vi "Dialog_parameters (SubVI).vi"() -> (3 "Cancelled?":bool)   [LabVIEW 2017]
doc: "Use this template to create a dialog box with event handling."
uses:
  Global_SNK3_HF.vi
  E:/_git/LV_Unicorn/LV_Unicorn.lvlib
panel:
  in  "TimerSyncInt":i32=10000 caption="Частота следования тактов, Гц" min=1000 max=100000
  in  "Meas":bool=TRUE
  in  "Tab2":T1(tab)
  in  "EncoderSync":i64=1 caption="Величина \"К\""
  out "NumOfRuns":i32=994875 caption="Счетчик количества запусков цикла"
  in  "DataEncodersParam2":enum16{"Encoder1CurrData", "PulseCurrData"}(ring) caption="Параметры поля \"Encoders Param 2\""
  in  "EncoderNum":u16(ring)=1 caption="Номер энкодера для режима \"Энкодер\"" items=["1"=1, "2"=2]
  in  "SyncMode":u16(ring)=1 caption="Источник синхронизации" items=["Внутренний таймер"=1, "Энкодер"=2, "Внешний импульс"=3]
  in  "DataEncodersParam1":enum16{"Encoder1CurrData", "PulseCurrData"}(ring) caption="Параметры поля \"Encoders Param 1\""
  in  "Encoder2CurrData":i64 caption="Текущее значение счетчика энкодера 2"
  in  "Encoder2ScalingFactor":i32=100 caption="Масштабный коэффициент, нм/имп"
  in  "Encoder2AInv":bool
  in  "Encoder2BInv":bool
  in  "Encoder2ZInv":bool
  in  "Encoder2ZEn":bool
  in  "Encoder2En":bool
  in  "Encoder1CurrData":i64 caption="Текущее значение счетчика энкодера 1"
  in  "Encoder1ScalingFactor":i32=100 caption="Масштабный коэффициент, нм/имп"
  in  "Encoder1AInv":bool
  in  "Encoder1BInv":bool
  in  "Encoder1ZInv":bool
  in  "Encoder1ZEn":bool
  in  "Encoder1En":bool
  in  "PulseCurrData":i64 caption="Текущее значение счетчика импульсов"
  in  "PulseSensitivity":u16(ring)=1 caption="Тип запуска для режима" items=["Фронт"=1, "Срез"=2, "Оба"=3]
  in  "PulseScalingFactor":i32=100 caption="Масштабный коэффициент, нм/имп" min=0
  in  "PulseInput":T2(ring) caption="Вход импульса запуска"
  in  "PulseCounterEn":bool
  in  "FPGA1ExtRAMBuffEn":bool=TRUE
  in  "FPGA0ExtRAMBuffEn":bool=TRUE
  in  "IPEn50Om":bool caption="Демпфирование ПЭП(50 Ом)"
  in  "ReceiverStaticGainParam":T3(ring) caption="Коэфф усиления приемников"
  in  "SaveParam":bool
  out "IPAddressCur":string caption="Текущий IP адрес ЭБ"
  in  "IPDefaultNetMask":string caption="Маска подсети"
  in  "IPDefaultGW":string caption="Основной шлюз"
  in  "IPDefaultAddress":string caption="IP адрес электронного блока по умолчанию"
  in  "IPAddressUDP":string caption="IP адрес для передачи UPD пакетов"
  in  "Port1UDP":u16 caption="Порт для передачи UPD пакетов с разъемов X1...X8"
  in  "Port2UDP":u16 caption="Порт для передачи UPD пакетов с разъемов X9...X16"
  in  "Cancel":bool
  in  "OK":bool
  # "Энкодер 1"
  # "Энкодер 2"
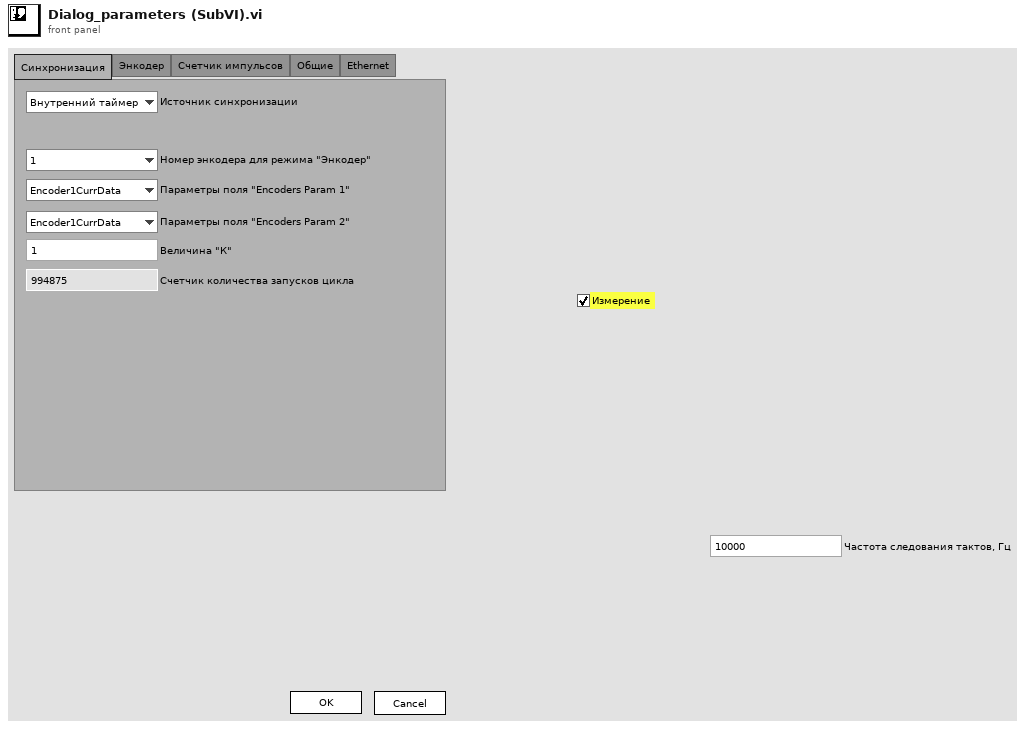
[diagram p1: front panel]
types:
  T1 = enum32{"Синхронизация", "Энкодер", "Счетчик импульсов", "Общие", "Ethernet"}
  T2 = enum16{"X17 вход 1", "X17 вход 2", "X17 вход 3", "X18 вход 1", "X18 вход 2", "X18 вход 3"}
  T3 = enum16{"Коэф. усил., дБ", "Вых. ЦАП (10 бит)", "Вых. ЦАП "}
  T4 = typedef "LV_Unicorn.lvlib/unicorn_Param.ctl" = cluster{"conParam":T5, "Param":T6}
  T5 = typedef "LV_Unicorn.lvlib/unicorn_conn.ctl" = cluster{"ReadIntParam":bool, "ReadDescrParam":bool, "ReadFloatParam":bool, "debug":bool, "ReadJSON":bool, "IP_address":string, "N_attempts":i32, "type_con":enum16{"Serial", "TCP"}, "MB_address":i32, "VISA":refnum<visa-resource-name>, "connection ID":refnum<k5>, "nameDevices":string, "timeout":i32, "port":u16, "type_version":string, "baud_rate":u32, "VersionControl":bool, "TCP_conn":bool, "WindowSize":i32}
  T6 = typedef "LV_Unicorn.lvlib/unicorn_JSON.ctl" = cluster{"NumParam":cluster{"NTelem":i32, "NInt":i32, "NFloat":i32, "NTable":i32}, "ParamInt":T7, "Telemetry":T8, "Table":T9, "ParamFloat":T10}
  T7 = typedef "LV_Unicorn.lvlib/unicorn_ParamInt.ctl" = cluster{"ID":string, "Num":i32, "Name":string, "Type":string, "Enum":string, "Desc":string, "Unit":string, "Access":string, "FormatStr":string, "Min":i32, "Max":i32}[]
  T8 = typedef "LV_Unicorn.lvlib/unicorn_Telemetry.ctl" = cluster{"ID":string, "Num":i32, "Name":string, "Desc":string, "Unit":string, "FormatStr":string, "Min":i32, "Max":i32}[]
  T9 = typedef "LV_Unicorn.lvlib/unicorn_Table.ctl" = cluster{"Num":i32, "Access":string, "ColumnCount":i32, "NeedParamPrepare":bool, "Columns":cluster{"Column":i32, "Desc":string, "Name":string}[], "DataType":string, "FormatStr":string, "ID":string, "Name":string, "RowCount":i32, "Rows":cluster{"Desc":string, "ID":string, "Max":i32, "Min":i32, "Name":string, "Row":i32, "Unit":string}[], "Type":string}[]
  T10 = typedef "LV_Unicorn.lvlib/unicorn_ParamFloat.ctl" = cluster{"ID":string, "Num":i32, "Name":string, "Type":string, "Enum":string, "Desc":string, "Unit":string, "Access":string, "FormatStr":string, "Min":sgl, "Max":sgl}[]
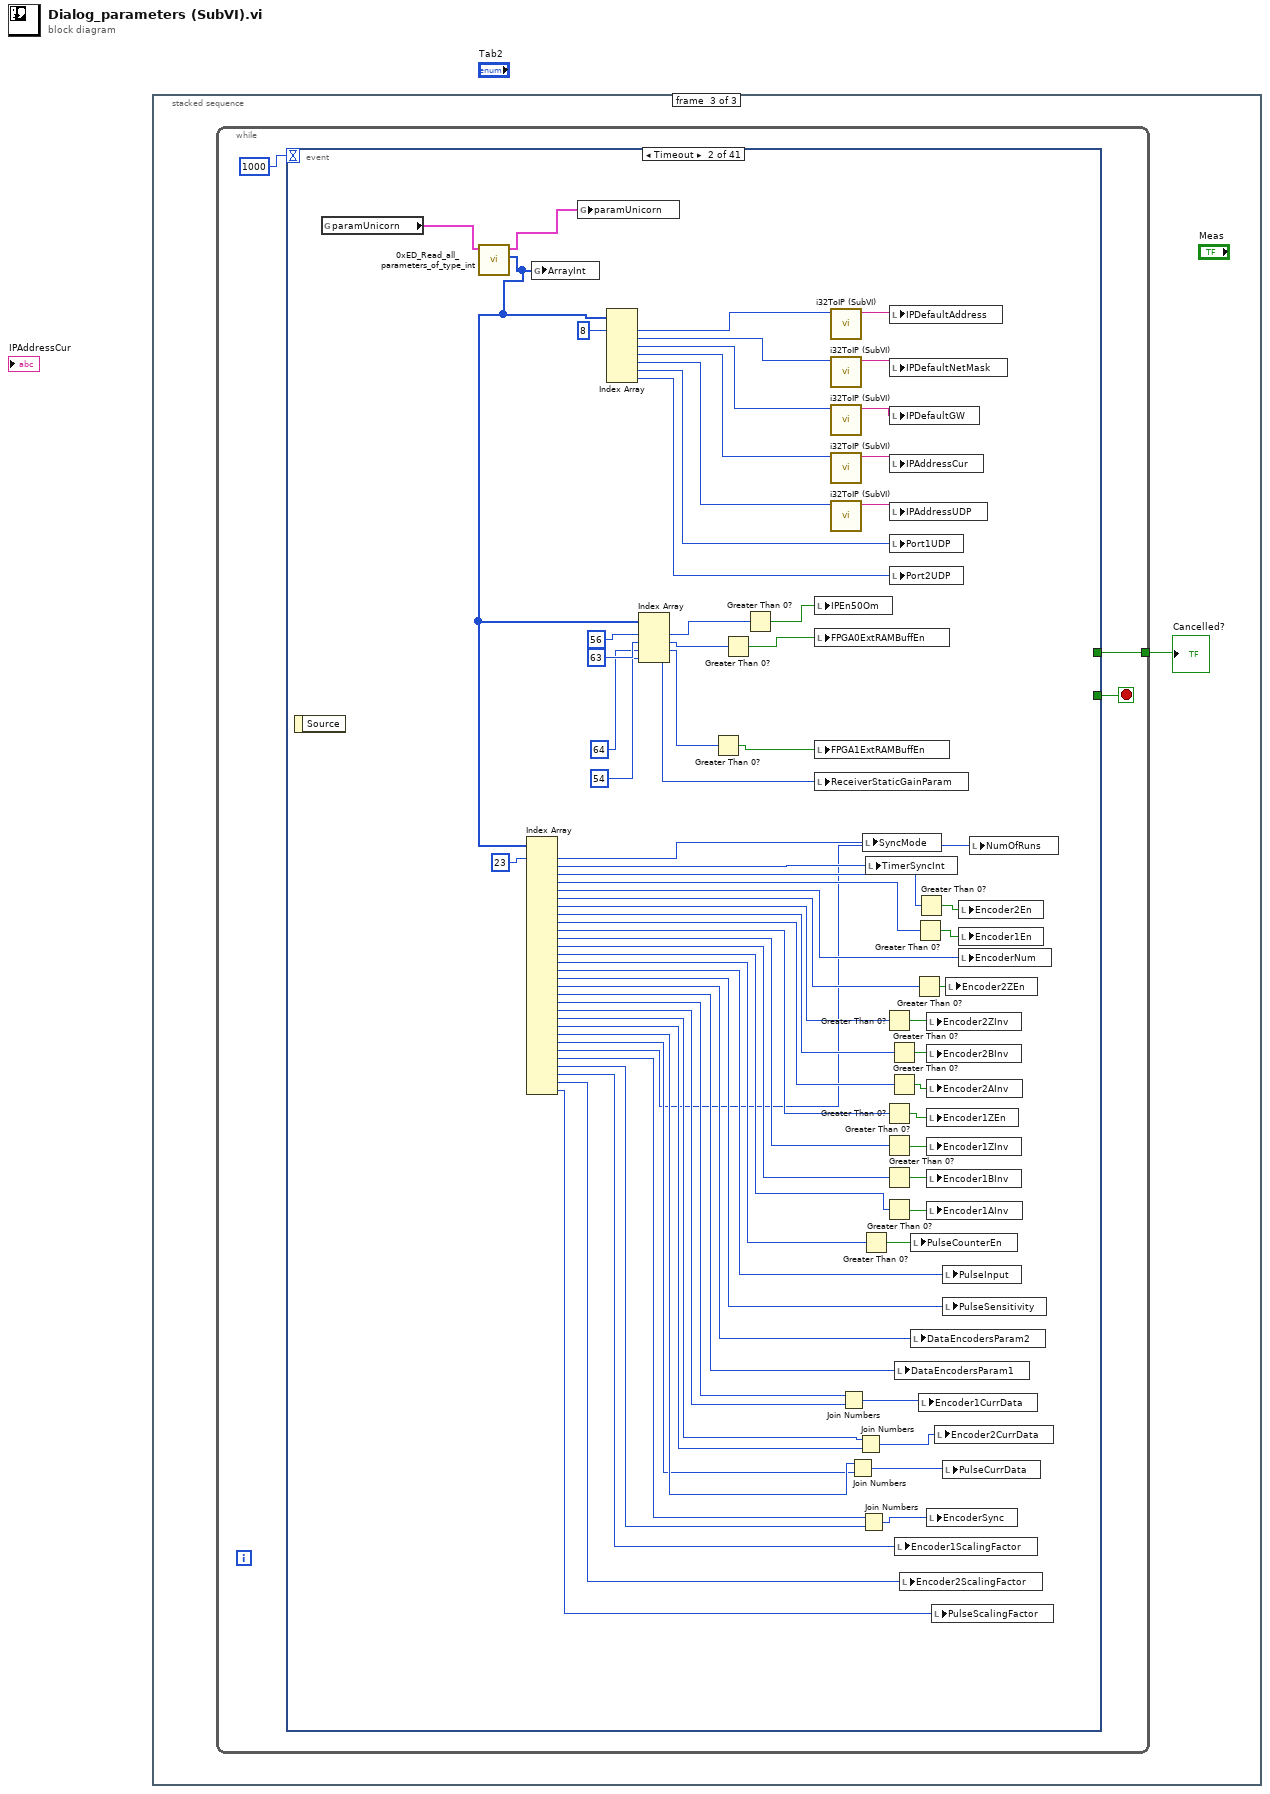
[diagram p0: block diagram]
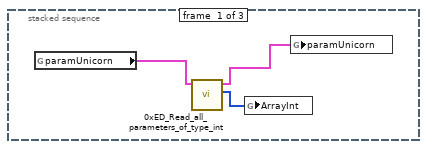
[diagram p2: hidden frame]
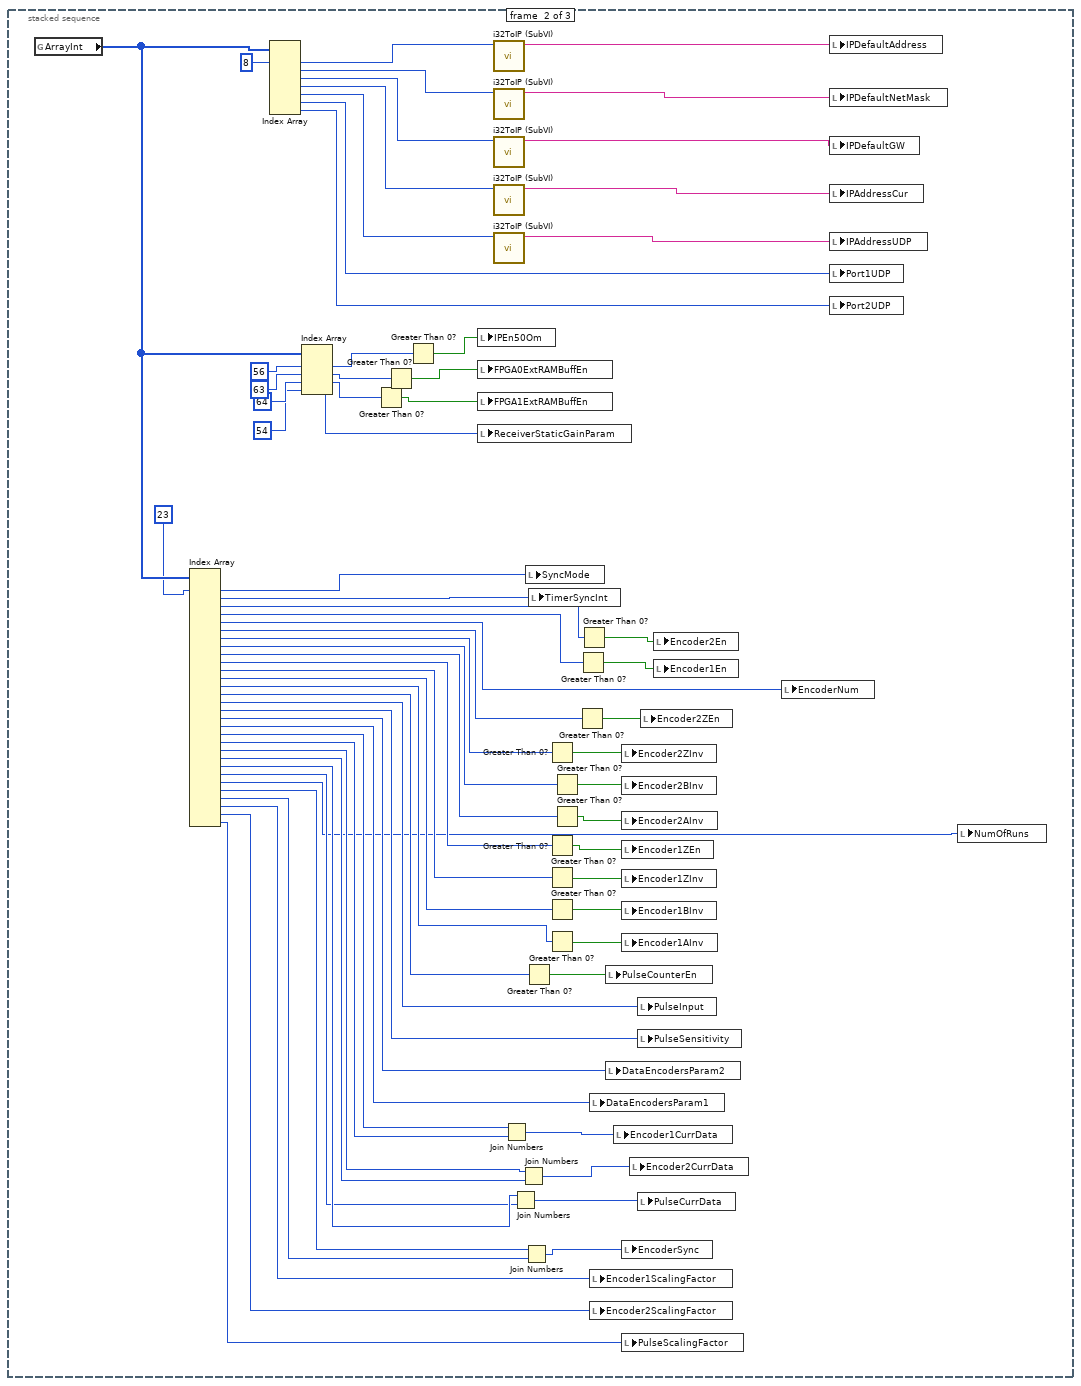
[diagram p3: hidden frame]
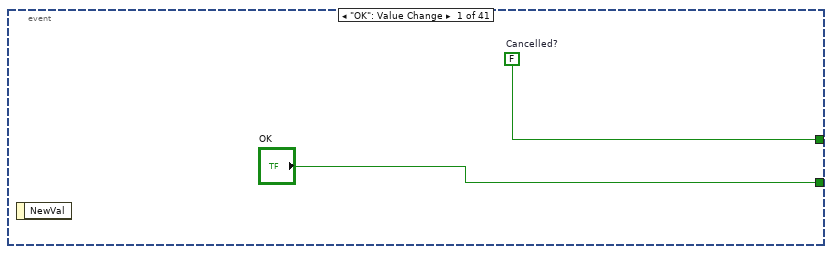
[diagram p4: hidden frame]
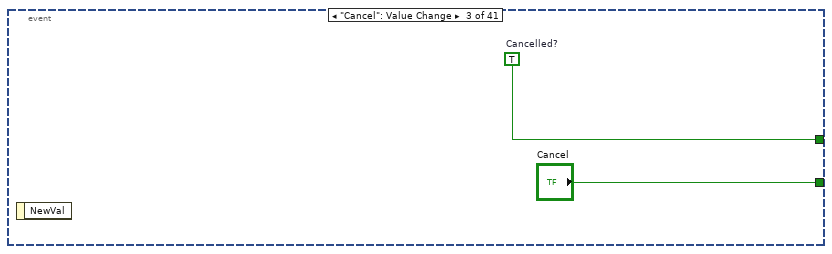
[diagram p5: hidden frame]
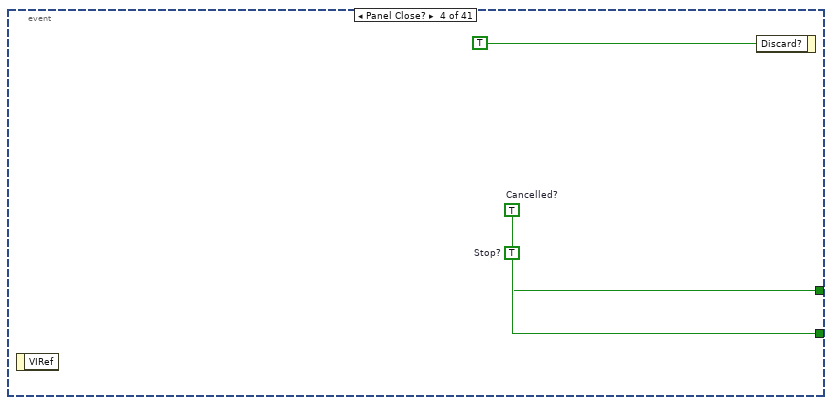
[diagram p6: hidden frame]
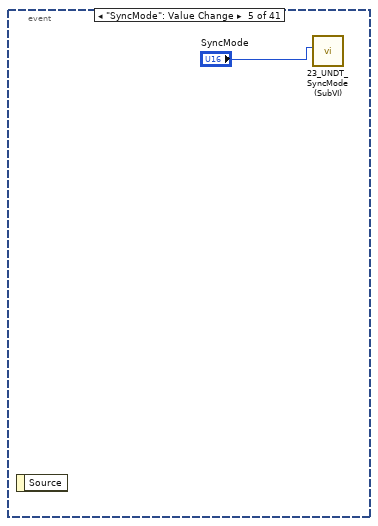
[diagram p7: hidden frame]
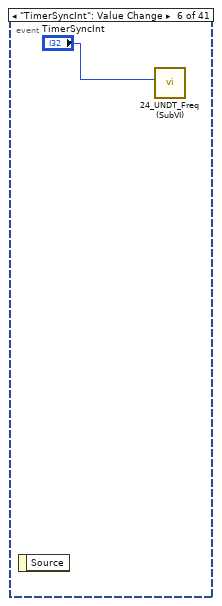
[diagram p8: hidden frame]
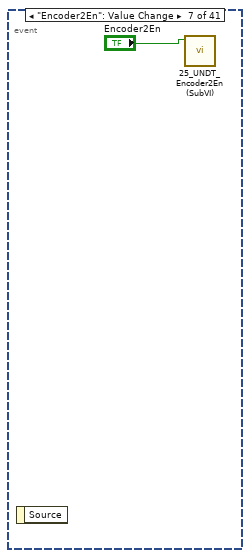
[diagram p9: hidden frame]
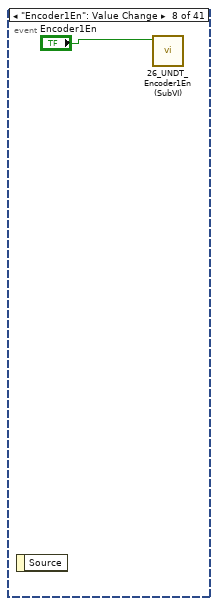
[diagram p10: hidden frame]
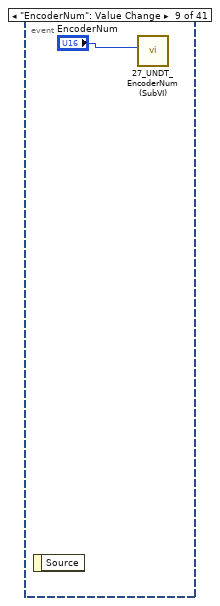
[diagram p11: hidden frame]
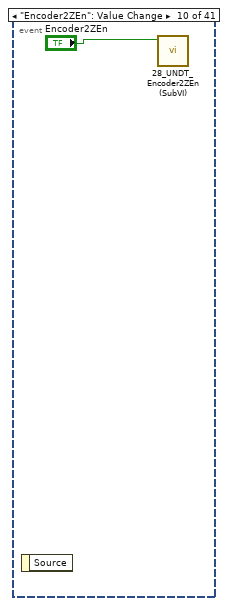
[diagram p12: hidden frame]
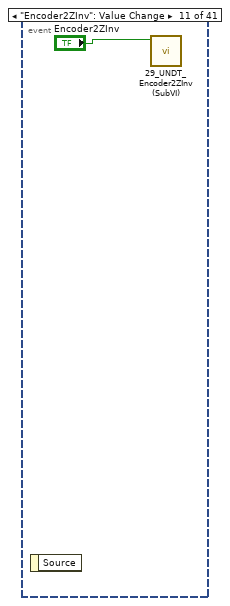
[diagram p13: hidden frame]
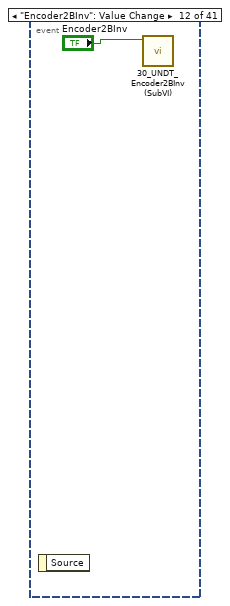
[diagram p14: hidden frame]
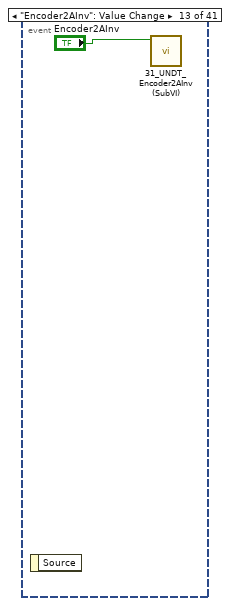
[diagram p15: hidden frame]
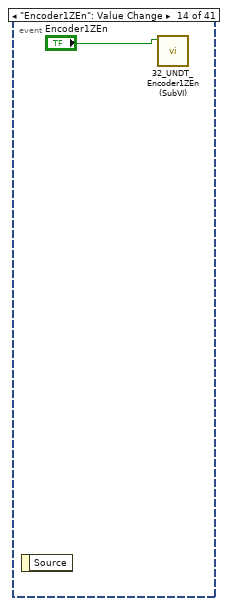
[diagram p16: hidden frame]
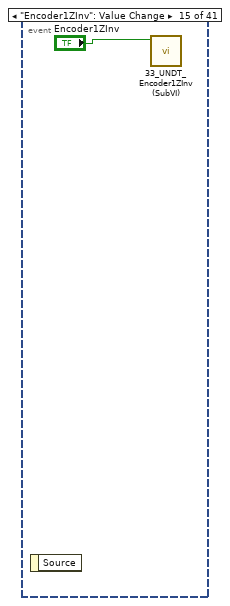
[diagram p17: hidden frame]
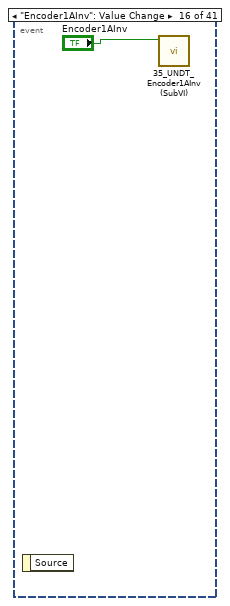
[diagram p18: hidden frame]
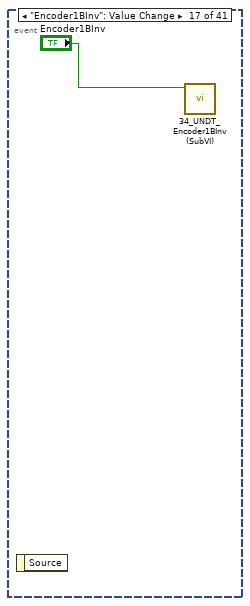
[diagram p19: hidden frame]
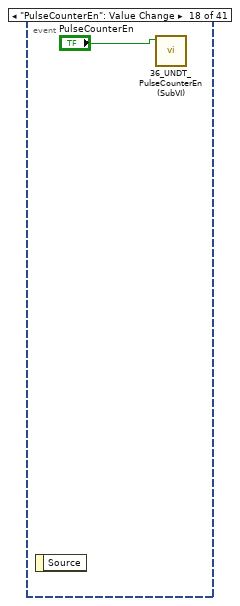
[diagram p20: hidden frame]
diagram:
  n1 = stacked-sequence {
    frame #0 {
      n2 = global read "Global_SNK3_HF.vi" "paramUnicorn"() -> (w3:T4)
      n3 = call "0xED_Read_all_parameters_of_type_int.vi"("paramUnicorn"=w3) -> ("ArrayInt"=w1:i32[], "paramUnicorn 2"=w2:T4)  [unwired: 7 in, 2 out]
      n4 = global write "Global_SNK3_HF.vi" "ArrayInt"(w1) -> ()
      n5 = global write "Global_SNK3_HF.vi" "paramUnicorn"(w2) -> ()
    }
    frame #1 {
      n6 = global read "Global_SNK3_HF.vi" "ArrayInt"() -> (w51:i32[])
      n7 = Index Array(array=w51, index #1=23 ("index")) -> (element #1=w43:i32, element #2=w41:i32, element #3=w40:i32, element #4=w39:i32, element #5=w38:i32, element #6=w35:i32, element #7=w47:i32, element #8=w46:i32, element #9=w45:i32, element #10=w30:i32, element #11=w29:i32, element #12=w28:i32, element #13=w27:i32, element #14=w26:i32, element #15=w24:i32, element #16=w23:i32, element #17=w22:i32, element #18=w21:i32, element #19=w20:i32, element #20=w19:i32, element #21=w17:i32, element #22=w16:i32, element #23=w14:i32, element #24=w13:i32, element #25=w11:i32, element #26=w9:i32, element #27=w8:i32, element #28=w7:i32, element #29=w6:i32, element #30=w5:i32)  [unwired: 29 in]
      n8 = Index Array(array=w51, index #1=8 ("index")) -> (element #1=w72:i32, element #2=w71:i32, element #3=w68:i32, element #4=w67:i32, element #5=w65:i32, element #6=w64:i32, element #7=w63:i32)  [unwired: 6 in]
      n9 = Index Array(array=w51, index #1=56 ("index"), index #2=63 ("index"), index #3=64 ("index"), index #4=54 ("index")) -> (element #1=w61:i32, element #2=w57:i32, element #3=w56:i32, element #4=w52:i32)
      n10 = Greater Than 0?(x=w56) -> (x > 0?=w54:bool)
      n11 = Greater Than 0?(x=w57) -> (x > 0?=w55:bool)
      n12 = Greater Than 0?(x=w61) -> (x > 0?=w60:bool)
      n13 = local write "IPEn50Om"(w60) -> ()
      n14 = local write "FPGA0ExtRAMBuffEn"(w55) -> ()
      n15 = local write "FPGA1ExtRAMBuffEn"(w54) -> ()
      n16 = local write "ReceiverStaticGainParam"(w52) -> ()
      n17 = call "i32ToIP (SubVI).vi"("int number"=w72) -> ("name"=w73:string)  [unwired: 10 in]
      n18 = call "i32ToIP (SubVI).vi"("int number"=w71) -> ("name"=w70:string)  [unwired: 10 in]
      n19 = call "i32ToIP (SubVI).vi"("int number"=w68) -> ("name"=w69:string)  [unwired: 10 in]
      n20 = call "i32ToIP (SubVI).vi"("int number"=w67) -> ("name"=w4:string)  [unwired: 10 in]
      n21 = call "i32ToIP (SubVI).vi"("int number"=w65) -> ("name"=w66:string)  [unwired: 10 in]
      n22 = Join Numbers(hi=w20, lo=w19) -> ((hi.lo)=w18:u64)
      n23 = Join Numbers(hi=w14, lo=w13) -> ((hi.lo)=w12:u64)
      n24 = Join Numbers(hi=w17, lo=w16) -> ((hi.lo)=w15:u64)
      n25 = Join Numbers(hi=w9, lo=w8) -> ((hi.lo)=w10:u64)
      n26 = Greater Than 0?(x=w26) -> (x > 0?=w25:bool)
      n27 = local write "SyncMode"(w43) -> ()
      n28 = local write "TimerSyncInt"(w41) -> ()
      n29 = Greater Than 0?(x=w47) -> (x > 0?=w37:bool)
      n30 = Greater Than 0?(x=w30) -> (x > 0?=w34:bool)
      n31 = Greater Than 0?(x=w29) -> (x > 0?=w33:bool)
      n32 = Greater Than 0?(x=w28) -> (x > 0?=w32:bool)
      n33 = Greater Than 0?(x=w27) -> (x > 0?=w31:bool)
      n34 = Greater Than 0?(x=w46) -> (x > 0?=w49:bool)
      n35 = Greater Than 0?(x=w45) -> (x > 0?=w48:bool)
      n36 = Greater Than 0?(x=w35) -> (x > 0?=w36:bool)
      n37 = Greater Than 0?(x=w39) -> (x > 0?=w42:bool)
      n38 = Greater Than 0?(x=w40) -> (x > 0?=w50:bool)
      n39 = local write "DataEncodersParam1"(w21) -> ()
      n40 = local write "Encoder1ScalingFactor"(w7) -> ()
      n41 = local write "Encoder2ScalingFactor"(w6) -> ()
      n42 = local write "PulseCounterEn"(w25) -> ()
      n43 = local write "DataEncodersParam2"(w22) -> ()
      n44 = local write "Encoder1CurrData"(w18) -> ()
      n45 = local write "Encoder2ZInv"(w37) -> ()
      n46 = local write "Encoder2BInv"(w49) -> ()
      n47 = local write "Encoder2AInv"(w48) -> ()
      n48 = local write "Encoder1ZEn"(w34) -> ()
      n49 = local write "Encoder1ZInv"(w33) -> ()
      n50 = local write "Encoder1BInv"(w32) -> ()
      n51 = local write "Encoder1AInv"(w31) -> ()
      n52 = local write "EncoderSync"(w10) -> ()
      n53 = local write "PulseScalingFactor"(w5) -> ()
      n54 = local write "Encoder2CurrData"(w15) -> ()
      n55 = local write "PulseInput"(w24) -> ()
      n56 = local write "PulseSensitivity"(w23) -> ()
      n57 = local write "PulseCurrData"(w12) -> ()
      n58 = local write "Encoder2ZEn"(w36) -> ()
      n59 = local write "Encoder2En"(w50) -> ()
      n60 = local write "Encoder1En"(w42) -> ()
      n61 = local write "EncoderNum"(w38) -> ()
      n62 = local write "IPDefaultAddress"(w73) -> ()
      n63 = local write "IPDefaultNetMask"(w70) -> ()
      n64 = local write "IPDefaultGW"(w69) -> ()
      n65 = local write "IPAddressCur"(w4) -> ()
      n66 = local write "IPAddressUDP"(w66) -> ()
      n67 = local write "Port1UDP"(w64) -> ()
      n68 = local write "Port2UDP"(w63) -> ()
      n69 = local write "NumOfRuns"(w11) -> ()
    }
    frame #2 {
      n70 = while {
        tunnel: [w77] -> w75
        stop <- w78 stop-if-true
        n71 = event shown="[1] Timeout" {
          selector: _ -> [_ _ _ _ _ _ _ _ _ _ _ _ _ _ _ _ _ _ _ _ _ _ _ _ _ _ _ _ _ _ _ _ _ _ _ _ _ _ _ _ _]
          dyn-events: _ -> [_ _ _ _ _ _ _ _ _ _ _ _ _ _ _ _ _ _ _ _ _ _ _ _ _ _ _ _ _ _ _ _ _ _ _ _ _ _ _ _ _]
          timeout: 1000 -> [_ _ _ _ _ _ _ _ _ _ _ _ _ _ _ _ _ _ _ _ _ _ _ _ _ _ _ _ _ _ _ _ _ _ _ _ _ _ _ _ _]
          tunnel: ["OK" _ "Cancel" w157 _ _ _ _ _ _ _ _ _ _ _ _ _ _ _ _ _ _ _ _ _ _ _ _ _ _ _ _ _ _ _ _ _ _ _ _ _] -> w78
          tunnel: [w80 _ w155 w156 _ _ _ _ _ _ _ _ _ _ _ _ _ _ _ _ _ _ _ _ _ _ _ _ _ _ _ _ _ _ _ _ _ _ _ _ _] -> w77
          event "OK": Value Change {
            w80 = FALSE  # Cancelled?
            n72 = event-data() -> ()  [unwired: 1 in, 1 out]
          }
          event Timeout {
            n73 = event-data() -> ()  [unwired: 1 in, 1 out]
            n74 = global read "Global_SNK3_HF.vi" "paramUnicorn"() -> (w153:T4)
            n75 = call "0xED_Read_all_parameters_of_type_int.vi"("paramUnicorn"=w153) -> ("ArrayInt"=w81:i32[], "paramUnicorn 2"=w152:T4)  [unwired: 7 in, 2 out]
            n76 = Index Array(array=w81, index #1=23 ("index")) -> (element #1=w127:i32, element #2=w125:i32, element #3=w124:i32, element #4=w123:i32, element #5=w122:i32, element #6=w119:i32, element #7=w130:i32, element #8=w129:i32, element #9=w128:i32, element #10=w114:i32, element #11=w113:i32, element #12=w112:i32, element #13=w111:i32, element #14=w110:i32, element #15=w108:i32, element #16=w107:i32, element #17=w106:i32, element #18=w105:i32, element #19=w104:i32, element #20=w103:i32, element #21=w101:i32, element #22=w100:i32, element #23=w98:i32, element #24=w97:i32, element #25=w95:i32, element #26=w93:i32, element #27=w92:i32, element #28=w91:i32, element #29=w90:i32, element #30=w89:i32)  [unwired: 29 in]
            n77 = global write "Global_SNK3_HF.vi" "ArrayInt"(w81) -> ()
            n78 = global write "Global_SNK3_HF.vi" "paramUnicorn"(w152) -> ()
            n79 = Index Array(array=w81, index #1=8 ("index")) -> (element #1=w150:i32, element #2=w149:i32, element #3=w146:i32, element #4=w145:i32, element #5=w143:i32, element #6=w142:i32, element #7=w141:i32)  [unwired: 6 in]
            n80 = Index Array(array=w81, index #1=56 ("index"), index #2=63 ("index"), index #3=64 ("index"), index #4=54 ("index")) -> (element #1=w140:i32, element #2=w138:i32, element #3=w137:i32, element #4=w134:i32)
            n81 = Greater Than 0?(x=w137) -> (x > 0?=w135:bool)
            n82 = Greater Than 0?(x=w138) -> (x > 0?=w136:bool)
            n83 = Greater Than 0?(x=w140) -> (x > 0?=w139:bool)
            n84 = local write "IPEn50Om"(w139) -> ()
            n85 = local write "FPGA0ExtRAMBuffEn"(w136) -> ()
            n86 = local write "FPGA1ExtRAMBuffEn"(w135) -> ()
            n87 = local write "ReceiverStaticGainParam"(w134) -> ()
            n88 = call "i32ToIP (SubVI).vi"("int number"=w150) -> ("name"=w151:string)  [unwired: 10 in]
            n89 = call "i32ToIP (SubVI).vi"("int number"=w149) -> ("name"=w148:string)  [unwired: 10 in]
            n90 = call "i32ToIP (SubVI).vi"("int number"=w146) -> ("name"=w147:string)  [unwired: 10 in]
            n91 = call "i32ToIP (SubVI).vi"("int number"=w145) -> ("name"=w88:string)  [unwired: 10 in]
            n92 = call "i32ToIP (SubVI).vi"("int number"=w143) -> ("name"=w144:string)  [unwired: 10 in]
            n93 = Join Numbers(hi=w104, lo=w103) -> ((hi.lo)=w102:u64)
            n94 = Join Numbers(hi=w98, lo=w97) -> ((hi.lo)=w96:u64)
            n95 = Join Numbers(hi=w101, lo=w100) -> ((hi.lo)=w99:u64)
            n96 = Join Numbers(hi=w93, lo=w92) -> ((hi.lo)=w94:u64)
            n97 = Greater Than 0?(x=w110) -> (x > 0?=w109:bool)
            n98 = local write "SyncMode"(w127) -> ()
            n99 = local write "TimerSyncInt"(w125) -> ()
            n100 = Greater Than 0?(x=w130) -> (x > 0?=w121:bool)
            n101 = Greater Than 0?(x=w114) -> (x > 0?=w118:bool)
            n102 = Greater Than 0?(x=w113) -> (x > 0?=w117:bool)
            n103 = Greater Than 0?(x=w112) -> (x > 0?=w116:bool)
            n104 = Greater Than 0?(x=w111) -> (x > 0?=w115:bool)
            n105 = Greater Than 0?(x=w129) -> (x > 0?=w132:bool)
            n106 = Greater Than 0?(x=w128) -> (x > 0?=w131:bool)
            n107 = local write "IPDefaultAddress"(w151) -> ()
            n108 = local write "IPDefaultNetMask"(w148) -> ()
            n109 = local write "IPDefaultGW"(w147) -> ()
            n110 = local write "IPAddressCur"(w88) -> ()
            n111 = local write "IPAddressUDP"(w144) -> ()
            n112 = local write "Port1UDP"(w142) -> ()
            n113 = local write "Port2UDP"(w141) -> ()
            n114 = local write "DataEncodersParam1"(w105) -> ()
            n115 = local write "Encoder1ScalingFactor"(w91) -> ()
            n116 = local write "Encoder2ScalingFactor"(w90) -> ()
            n117 = local write "PulseCounterEn"(w109) -> ()
            n118 = local write "DataEncodersParam2"(w106) -> ()
            n119 = Greater Than 0?(x=w119) -> (x > 0?=w120:bool)
            n120 = Greater Than 0?(x=w123) -> (x > 0?=w126:bool)
            n121 = Greater Than 0?(x=w124) -> (x > 0?=w133:bool)
            n122 = local write "Encoder1CurrData"(w102) -> ()
            n123 = local write "Encoder2ZInv"(w121) -> ()
            n124 = local write "Encoder2BInv"(w132) -> ()
            n125 = local write "Encoder2AInv"(w131) -> ()
            n126 = local write "Encoder1ZEn"(w118) -> ()
            n127 = local write "Encoder1ZInv"(w117) -> ()
            n128 = local write "Encoder1BInv"(w116) -> ()
            n129 = local write "Encoder1AInv"(w115) -> ()
            n130 = local write "EncoderSync"(w94) -> ()
            n131 = local write "PulseScalingFactor"(w89) -> ()
            n132 = local write "Encoder2CurrData"(w99) -> ()
            n133 = local write "PulseInput"(w108) -> ()
            n134 = local write "PulseSensitivity"(w107) -> ()
            n135 = local write "PulseCurrData"(w96) -> ()
            n136 = local write "Encoder2ZEn"(w120) -> ()
            n137 = local write "Encoder2En"(w133) -> ()
            n138 = local write "Encoder1En"(w126) -> ()
            n139 = local write "EncoderNum"(w122) -> ()
            n140 = local write "NumOfRuns"(w95) -> ()
          }
          event "Cancel": Value Change {
            w155 = TRUE  # Cancelled?
            n141 = event-data() -> ()  [unwired: 1 in, 1 out]
          }
          event Panel Close? {
            w156 = TRUE  # Cancelled?
            w157 = TRUE  # Stop?
            n142 = event-data() -> ()  [unwired: 1 in, 1 out]
            n143 = event-data("Discard?"=TRUE) -> ()  [unwired: 1 in, 1 out]
          }
          event "SyncMode": Value Change {
            n144 = event-data() -> ()  [unwired: 1 in, 1 out]
            n145 = call "23_UNDT_SyncMode (SubVI).vi"("SyncMode"="SyncMode") -> ()  [unwired: 10 in, 1 out]
          }
          event "TimerSyncInt": Value Change {
            n146 = event-data() -> ()  [unwired: 1 in, 1 out]
            n147 = call "24_UNDT_Freq (SubVI).vi"("UNDT_Freq"="TimerSyncInt") -> ()  [unwired: 10 in, 1 out]
          }
          event "Encoder2En": Value Change {
            n148 = event-data() -> ()  [unwired: 1 in, 1 out]
            n149 = call "25_UNDT_Encoder2En (SubVI).vi"("Encoder2En"="Encoder2En") -> ()  [unwired: 9 in, 2 out]
          }
          event "Encoder1En": Value Change {
            n150 = event-data() -> ()  [unwired: 1 in, 1 out]
            n151 = call "26_UNDT_Encoder1En (SubVI).vi"("Encoder1En"="Encoder1En") -> ()  [unwired: 9 in, 2 out]
          }
          event "EncoderNum": Value Change {
            n152 = event-data() -> ()  [unwired: 1 in, 1 out]
            n153 = call "27_UNDT_EncoderNum (SubVI).vi"("EncoderNum"="EncoderNum") -> ()  [unwired: 10 in, 1 out]
          }
          event "Encoder2ZEn": Value Change {
            n154 = event-data() -> ()  [unwired: 1 in, 1 out]
            n155 = call "28_UNDT_Encoder2ZEn (SubVI).vi"("Encoder2ZEn"="Encoder2ZEn") -> ()  [unwired: 9 in, 2 out]
          }
          event "Encoder2ZInv": Value Change {
            n156 = event-data() -> ()  [unwired: 1 in, 1 out]
            n157 = call "29_UNDT_Encoder2ZInv (SubVI).vi"("Encoder2ZInv"="Encoder2ZInv") -> ()  [unwired: 9 in, 2 out]
          }
          event "Encoder2BInv": Value Change {
            n158 = event-data() -> ()  [unwired: 1 in, 1 out]
            n159 = call "30_UNDT_Encoder2BInv (SubVI).vi"("Encoder2BInv"="Encoder2BInv") -> ()  [unwired: 9 in, 2 out]
          }
          event "Encoder2AInv": Value Change {
            n160 = event-data() -> ()  [unwired: 1 in, 1 out]
            n161 = call "31_UNDT_Encoder2AInv (SubVI).vi"("Encoder2AInv"="Encoder2AInv") -> ()  [unwired: 9 in, 2 out]
          }
          event "Encoder1ZEn": Value Change {
            n162 = event-data() -> ()  [unwired: 1 in, 1 out]
            n163 = call "32_UNDT_Encoder1ZEn (SubVI).vi"("Encoder1ZEn"="Encoder1ZEn") -> ()  [unwired: 9 in, 2 out]
          }
          event "Encoder1ZInv": Value Change {
            n164 = event-data() -> ()  [unwired: 1 in, 1 out]
            n165 = call "33_UNDT_Encoder1ZInv (SubVI).vi"("Encoder1ZInv"="Encoder1ZInv") -> ()  [unwired: 9 in, 2 out]
          }
          event "Encoder1AInv": Value Change {
            n166 = event-data() -> ()  [unwired: 1 in, 1 out]
            n167 = call "35_UNDT_Encoder1AInv (SubVI).vi"("Encoder1AInv"="Encoder1AInv") -> ()  [unwired: 9 in, 2 out]
          }
          event "Encoder1BInv": Value Change {
            n168 = event-data() -> ()  [unwired: 1 in, 1 out]
            n169 = call "34_UNDT_Encoder1BInv (SubVI).vi"("Encoder1BInv"="Encoder1BInv") -> ()  [unwired: 9 in, 2 out]
          }
          event "PulseCounterEn": Value Change {
            n170 = event-data() -> ()  [unwired: 1 in, 1 out]
            n171 = call "36_UNDT_PulseCounterEn (SubVI).vi"("PulseCounterEn"="PulseCounterEn") -> ()  [unwired: 9 in, 2 out]
          }
          event "PulseInput": Value Change {
            n172 = event-data() -> ()  [unwired: 1 in, 1 out]
            n173 = call "37_UNDT_PulseInput (SubVI).vi"("PulseInput"="PulseInput") -> ()  [unwired: 10 in, 1 out]
          }
          event "PulseSensitivity": Value Change {
            n174 = event-data() -> ()  [unwired: 1 in, 1 out]
            n175 = call "38_UNDT_PulseSensitivity (SubVI).vi"("PulseSensitivity"="PulseSensitivity") -> ()  [unwired: 10 in, 1 out]
          }
          event "DataEncodersParam2": Value Change {
            n176 = event-data() -> ()  [unwired: 1 in, 1 out]
            n177 = call "39_UNDT_PulseCurrData (SubVI).vi"("DataEncodersParam2"="DataEncodersParam2") -> ()  [unwired: 10 in, 1 out]
          }
          event "DataEncodersParam1": Value Change {
            n178 = event-data() -> ()  [unwired: 1 in, 1 out]
            n179 = call "40_UNDT_DataEncodersParam1 (SubVI).vi"("DataEncodersParam1"="DataEncodersParam1") -> ()  [unwired: 10 in, 1 out]
          }
          event "Encoder1CurrData": Value Change {
            n180 = event-data() -> ()  [unwired: 1 in, 1 out]
            n181 = call "41_42_UNDT_Encoder1CurrData (SubVI).vi"("Encoder1CurrData"="Encoder1CurrData") -> ()  [unwired: 10 in, 1 out]
          }
          event "Encoder2CurrData": Value Change {
            n182 = event-data() -> ()  [unwired: 1 in, 1 out]
            n183 = call "43_44_UNDT_Encoder2CurrData (SubVI).vi"("Encoder2CurrData"="Encoder2CurrData") -> ()  [unwired: 10 in, 1 out]
          }
          event "PulseCurrData": Value Change {
            n184 = event-data() -> ()  [unwired: 1 in, 1 out]
            n185 = call "45_46_UNDT_PulseCurrDataH (SubVI).vi"("PulseCurrData"="PulseCurrData") -> ()  [unwired: 10 in, 1 out]
          }
          event "NumOfRuns": Value Change {
            n186 = event-data() -> ()  [unwired: 1 in, 1 out]
            n187 = disable-structure shown="Disabled" {
              frame Disabled {
                n188 = call "47_UNDT_NumOfRuns (SubVI).vi"() -> ("NumOfRuns"=→"NumOfRuns":i32)  [unwired: 10 in, 1 out]
              }
              frame Enabled {
              }
            }
          }
          event "EncoderSync": Value Change {
            n189 = event-data() -> ()  [unwired: 1 in, 1 out]
            n190 = call "48_49_UNDT_Encoder2CurrData (SubVI).vi"("EncoderSync"="EncoderSync") -> ()  [unwired: 10 in, 1 out]
          }
          event "Encoder1ScalingFactor": Value Change {
            n191 = event-data() -> ()  [unwired: 1 in, 1 out]
            n192 = call "50_UNDT_Encoder1ScalingFactor (SubVI).vi"("Encoder1ScalingFactor"="Encoder1ScalingFactor") -> ()  [unwired: 10 in, 1 out]
          }
          event "Encoder2ScalingFactor": Value Change {
            n193 = event-data() -> ()  [unwired: 1 in, 1 out]
            n194 = call "51_UNDT_Encoder1ScalingFactor (SubVI).vi"("Encoder2ScalingFactor"="Encoder2ScalingFactor") -> ()  [unwired: 10 in, 1 out]
          }
          event "PulseScalingFactor": Value Change {
            n195 = event-data() -> ()  [unwired: 1 in, 1 out]
            n196 = call "52_UNDT_PulseScalingFactor (SubVI).vi"("PulseScalingFactor"="PulseScalingFactor") -> ()  [unwired: 10 in, 1 out]
          }
          event "FPGA0ExtRAMBuffEn": Value Change {
            n197 = event-data() -> ()  [unwired: 1 in, 1 out]
            n198 = call "63_UNDT_FPGA0ExtRAMBuffEn (SubVI).vi"("FPGA0ExtRAMBuffEn"="FPGA0ExtRAMBuffEn") -> ()  [unwired: 9 in, 2 out]
          }
          event "FPGA1ExtRAMBuffEn": Value Change {
            n199 = event-data() -> ()  [unwired: 1 in, 1 out]
            n200 = call "64_UNDT_FPGA1ExtRAMBuffEn (SubVI).vi"("FPGA1ExtRAMBuffEn"="FPGA1ExtRAMBuffEn") -> ()  [unwired: 10 in, 1 out]
          }
          event "IPDefaultNetMask": Value Change {
            n201 = event-data() -> ()  [unwired: 1 in, 1 out]
            n202 = call "09_UNDT_IPDefaultNetMask (SubVI).vi"("IPDefaultNetMask"="IPDefaultNetMask") -> ()  [unwired: 10 in, 1 out]
          }
          event "IPDefaultGW": Value Change {
            n203 = event-data() -> ()  [unwired: 1 in, 1 out]
            n204 = call "10_UNDT_IPDefaultGW (SubVI).vi"("IPDefaultGW"="IPDefaultGW") -> ()  [unwired: 10 in, 1 out]
          }
          event "IPDefaultAddress": Value Change {
            n205 = event-data() -> ()  [unwired: 1 in, 1 out]
            n206 = call "08_UNDT_IPDefaultAddress (SubVI).vi"("IPDefaultAddress"="IPDefaultAddress") -> ()  [unwired: 10 in, 1 out]
          }
          event "IPAddressUDP": Value Change {
            n207 = event-data() -> ()  [unwired: 1 in, 1 out]
            n208 = call "12_UNDT_IPAddressUDP (SubVI).vi"("IP_PC"="IPAddressUDP") -> ()  [unwired: 10 in, 1 out]
          }
          event "Port1UDP": Value Change {
            n209 = event-data() -> ()  [unwired: 1 in, 1 out]
            n210 = call "13_UNDT_Port1UDP (SubVI).vi"("Port1UDP"="Port1UDP") -> ()  [unwired: 10 in, 1 out]
          }
          event "Port2UDP": Value Change {
            n211 = event-data() -> ()  [unwired: 1 in, 1 out]
            n212 = call "14_UNDT_Port2UDP (SubVI).vi"("Port2UDP"="Port2UDP") -> ()  [unwired: 10 in, 1 out]
          }
          event "IPEn50Om": Value Change {
            n213 = event-data() -> ()  [unwired: 1 in, 1 out]
            n214 = call "56_UNDT_IPEn50Om (SubVI).vi"("IPEn50Om"="IPEn50Om") -> ()  [unwired: 9 in, 2 out]
          }
          event "ReceiverStaticGainParam": Value Change {
            # "54 параметр определяющий коэфф усиления приемников"
            n215 = event-data() -> ()  [unwired: 1 in, 1 out]
            n216 = call "NotUse_54_UNDT_ReceiverStaticGainParam (SubVI).vi"("ReceiverStaticGainParam"="ReceiverStaticGainParam") -> ()  [unwired: 10 in, 1 out]
          }
          event "SaveParam": Value Change {
            n217 = event-data() -> ()  [unwired: 1 in, 1 out]
            n218 = stacked-sequence {
              frame #0 {
              }
              frame #1 {
                n219 = call "22_UNDT_IPSaveParam (SubVI).vi"() -> ("Значение параметра"=w196:i32)  [unwired: 10 in, 1 out]
                n220 = case shown="1, Default" w196 {
                  tunnel: ["Параметры сохранены в FLASH память ЭБ." ("message") "Сохранение невыполнено!" ("message")] -> w195
                  frame 0 {
                  }
                  frame 1, Default {
                  }
                }
                n221 = One Button Dialog(message=w195) -> ()  [unwired: 1 in, 1 out]
              }
            }
          }
        }
      }
      "Cancelled?" <- w75
    }
  }
